vi "Get SDK Version.vi"(8 "error in (no error)":errorcluster) -> (0 "error out":errorcluster, 2 "Version":string, 3 "Result":i32)   [LabVIEW 2018, in "Fujifilm X Series GFX System Digital Camera.lvlib"]
doc: "Gets version numbers in a string format."
uses:
  <instrlib>/Fujifilm X Series GFX System Digital Camera/Fujifilm X Series GFX System Digital Camera.lvlib
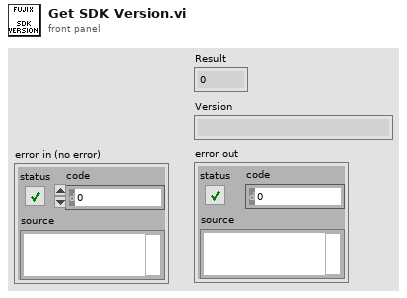
[diagram p1: front panel]
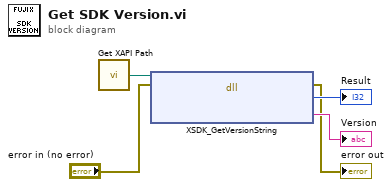
[diagram p0: block diagram]
diagram:
  n1 = call <instrlib>:"Get XAPI Path.vi"() -> ("XAPI Library Path"=w5:path)  [unwired: 1 in]
  n2 = dll-call lib="?" fn="XSDK_GetVersionString"(path in=w5, error in="error in (no error)") -> (error out=→"error out":errorcluster, "return type"=→"Result":i32, "pVersionString"=→"Version":string)  [unwired: 2 in, 1 out]
